vi "Runtime Test.vi"() -> ()   [LabVIEW 2014, in "DAQmx Watchdog tests.lvlib"]
uses:
  DAQmx Watchdog tests.lvlib
  module/execution/DAQmx Watchdog runtime.lvclass
  <vilib>/NI/Tag Bus/dictionary/data dictionary.lvclass/data dictionary.ctl
  <vilib>/NI/Tag Bus/dictionary/lookup polymorphs/locate Boolean.vi
  <vilib>/NI/Tag Bus/table/data polymorphs/read one/read Boolean.vi
  <vilib>/NI/Tag Bus/table/data polymorphs/write one/write Boolean.vi
  <vilib>/NI/Tag Bus/dictionary/search/find data index.vi
  <vilib>/NI/Tag Bus/dictionary/search/search string list.vi
  <vilib>/NI/Tag Bus/dictionary/tag not found.vi
  module/configuration/DAQmx Watchdog configuration.lvclass
  <vilib>/NI/Tag Bus/dictionary/data dictionary.lvclass
  <vilib>/NI/Tag Bus/table/data table.lvlib
panel:
  out "Expired?":bool
  out "input lookup error":errorcluster
  out "input error":errorcluster
  out "process result lookup error":errorcluster
  out "final error":errorcluster
  out "output error":errorcluster
  out "process error":errorcluster
  out "output lookup error":errorcluster
  out "process parameter  lookup error":errorcluster
  out "correct execution settings":bool
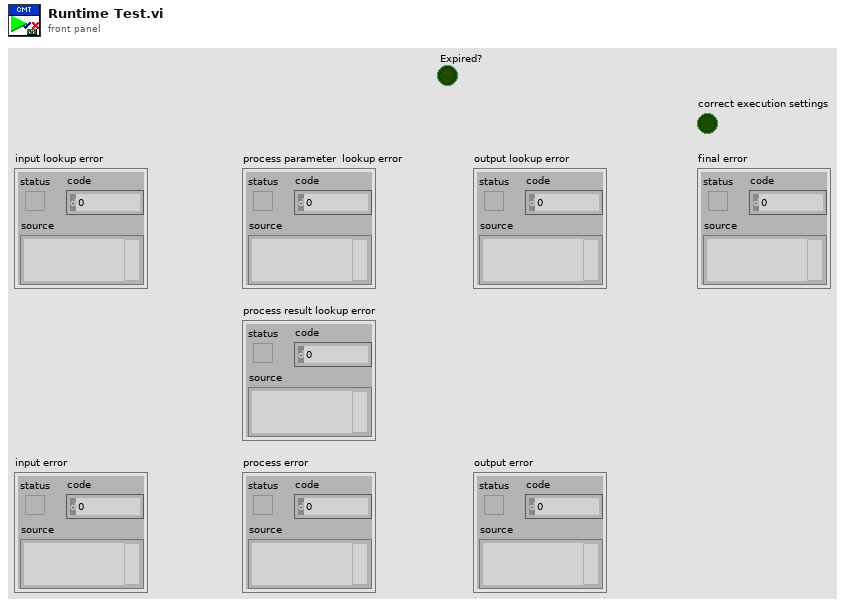
[diagram p1: front panel]
types:
  T1 = typedef "TBM channel.lvclass/data tables.ctl" = cluster{"input data":T2, "processing parameter":T2, "processing result":T2, "output data":T2}
  T2 = typedef "tag bus.lvlib/dictionary table pair.ctl" = cluster{"data dictionary":refnum<class "data dictionary.lvclass">, "data table":T3}
  T3 = typedef "tag bus.lvlib/data table.lvlib/data table.ctl" = cluster{"Double":dbl[], "Single":sgl[], "I64":i64[], "I32":i32[], "I16":i16[], "I8":i8[], "U64":u64[], "U32":u32[], "U16":u16[], "U8":u8[], "Boolean":bool[], "String":string[], "Array of Double":cluster{"DBL Array":dbl[]}[], "Array of Single":cluster{"SGL Array":sgl[]}[], "Array of I64":cluster{"I64 Array":i64[]}[], "Array of I32":cluster{"I32 Array":i32[]}[], "Array of I16":cluster{"I16 Array":i16[]}[], "Array of I8":cluster{"I8 Array":i8[]}[], "Array of U64":cluster{"U64 Array":u64[]}[], "Array of U32":cluster{"U32 Array":u32[]}[], "Array of U16":cluster{"U16 Array":u16[]}[], "Array of U8":cluster{"U8 Array":u8[]}[], "Array of Boolean":cluster{"Boolean Array":bool[]}[], "Array of String":cluster{"String Array":string[]}[]}
  T4 = typedef "TBM module execution interface.lvclass/execution settings.ctl" = cluster{"reads inputs":bool, "processes data":bool, "writes outputs":bool}
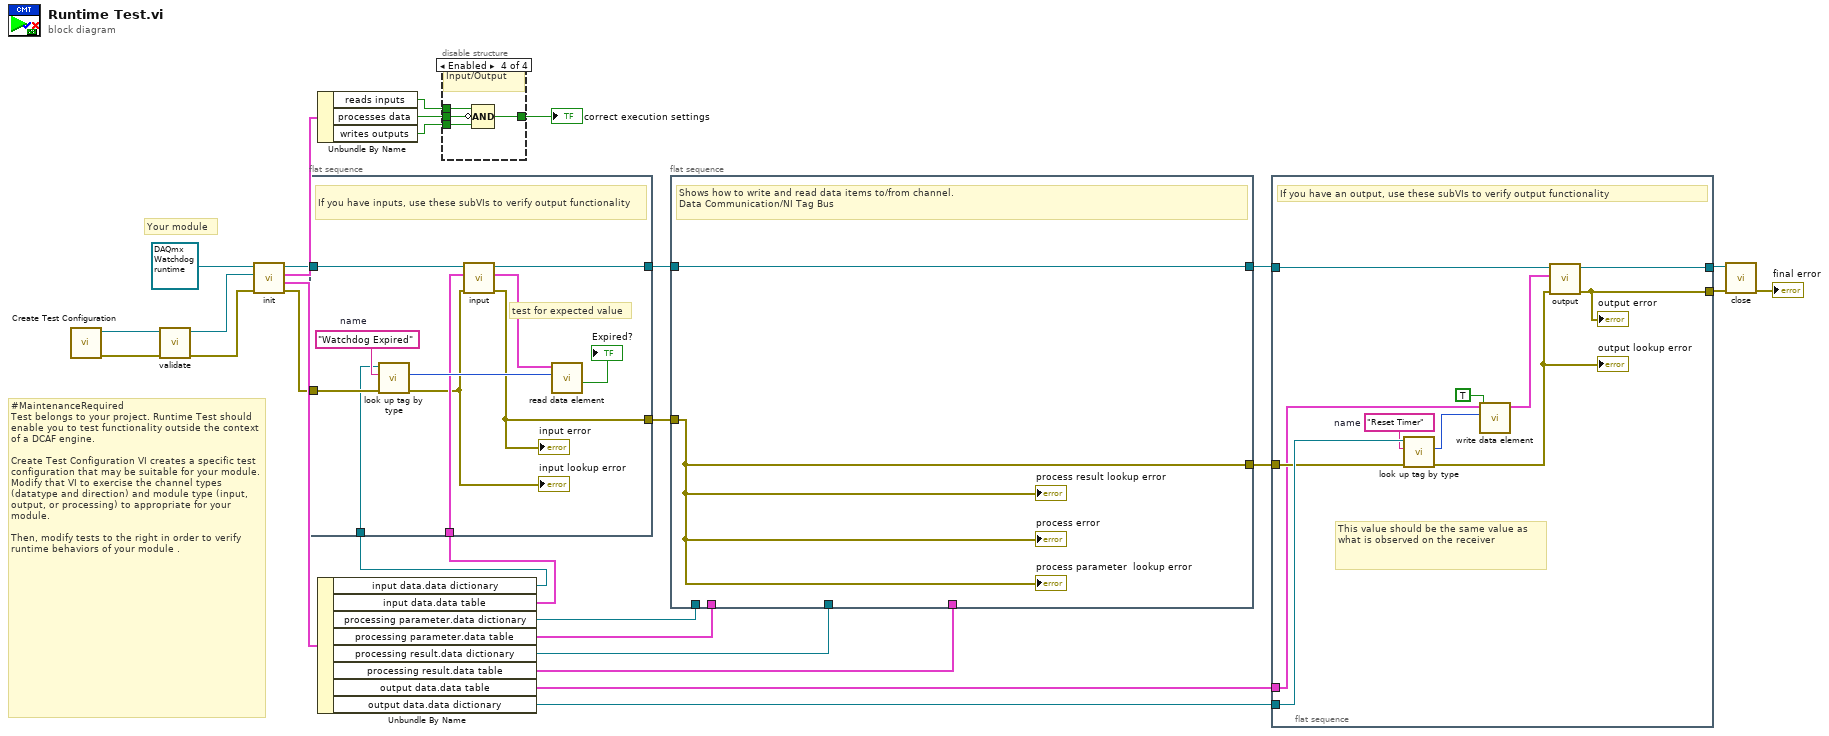
[diagram p0: block diagram]
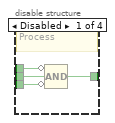
[diagram p2: hidden frame]
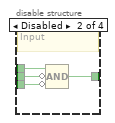
[diagram p3: hidden frame]
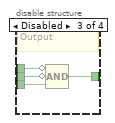
[diagram p4: hidden frame]
diagram:
  # "Your module"
  # "#MaintenanceRequired\nTest belongs to your project. Runtime Test should enable you to test functionality outside the context of a DCAF engine. \n\nCreate Test Configuration VI creates a specific test configuration that may be suitable for your module. Modify that VI to exercise the channel types (datatype and direction) and module type (input, output, or processing) to appropriate for your module. \n\nThen, modify tests to the right in order to verify runtime behaviors of your module ."
  n1 = call "Create Test Configuration.vi"() -> ("error out"=w9:errorcluster, "Module"=w11:refnum<class "DAQmx Watchdog configuration.lvclass">)  [unwired: 6 in, 4 out]
  n2 = call-dynamic "validate.vi"("error in"=w9, "fixed channel configuration in"=w11) -> ("error out"=w27:errorcluster, "fixed channel configuration out"=w28:refnum<class "DAQmx Watchdog configuration.lvclass">)  [unwired: 8 in]
  n3 = call-dynamic "init.vi"("error in"=w27, "TBM module configuration in"=w28, "fixed channel runtime in"=refnum<class "DAQmx Watchdog runtime.lvclass"> refnum ("user module")) -> ("error out"=w8:errorcluster, "data allocations"=w22:T1, "execution settings"=w26:T4, "fixed channel runtime out"=w6:refnum<class "DAQmx Watchdog runtime.lvclass">)  [unwired: 5 in]
  n4 = flat-sequence {
    tunnel: w8 -> [w36]
    tunnel: [w31] -> w7
    tunnel: w6 -> [w39]
    tunnel: [w38] -> w5
    tunnel: w4 -> [w35]
    tunnel: w1 -> [w32]
    frame #0 {
      w37 = "Watchdog Expired"  # name
      # "test for expected value"
      # "If you have inputs, use these subVIs to verify output functionality"
      n5 = call-poly <vilib>:"look up tag by type.vi"("error in"=w36, "name"=w37, "data dictionary in"=w35) -> ("error out"=w30:errorcluster, "index"=w33:i32)  [unwired: 6 in, 1 out]
      "input lookup error" <- w30
      n6 = call-dynamic "input.vi"("error in"=w30, "input allocation"=w32, "DAQmx Watchdog runtime in"=w39) -> ("error out"=w31:errorcluster, "input data"=w34:T3, "DAQmx Watchdog runtime out"=w38:refnum<class "DAQmx Watchdog runtime.lvclass">)  [unwired: 6 in]
      "input error" <- w31
      n7 = call-poly <vilib>:"read data element.vi"("index"=w33, "data table in"=w34) -> ("value"=→"Expired?":bool)  [unwired: 8 in, 1 out]
    }
  }
  n8 = Unbundle By Name(w26) -> ("reads inputs"=w24:bool, "processes data"=w12:bool, "writes outputs"=w25:bool)
  n9 = Unbundle By Name(w22) -> ("input data.data dictionary"=w4:refnum<class "data dictionary.lvclass">, "input data.data table"=w1:T3, "processing parameter.data dictionary"=w21:refnum<class "data dictionary.lvclass">, "processing parameter.data table"=w20:T3, "processing result.data dictionary"=w3:refnum<class "data dictionary.lvclass">, "processing result.data table"=w2:T3, "output data.data table"=w13:T3, "output data.data dictionary"=w19:refnum<class "data dictionary.lvclass">)
  n10 = disable-structure shown="Enabled" {
    disable-tunnel: w25 -> [w43 w47 w51 w55]
    disable-tunnel: w24 -> [w42 w46 w50 w54]
    disable-tunnel: [w41 w45 w49 w53] -> w23
    disable-tunnel: w12 -> [w40 w44 w48 w52]
    frame Disabled {
      # "Process"
      n11 = Compound Arithmetic op=AND(invert w42, w40, invert w43) -> (w41:bool)
    }
    frame Disabled {
      # "Input"
      n12 = Compound Arithmetic op=AND(w46, invert w44, invert w47) -> (w45:bool)
    }
    frame Disabled {
      # "Output"
      n13 = Compound Arithmetic op=AND(invert w50, invert w48, w51) -> (w49:bool)
    }
    frame Enabled {
      # "Input/Output"
      n14 = Compound Arithmetic op=AND(w54, invert w52, w55) -> (w53:bool)
    }
  }
  "correct execution settings" <- w23
  n15 = flat-sequence {
    tunnel: w21 -> [_]
    tunnel: w7 -> [w56]
    tunnel: w20 -> [_]
    tunnel: [w57] -> w15
    tunnel: [w56] -> w14
    tunnel: w5 -> [w57]
    tunnel: w3 -> [_]
    tunnel: w2 -> [_]
    frame #0 {
      # "Shows how to write and read data items to/from channel.\nData Communication/NI Tag Bus"
      "process parameter  lookup error" <- w56
      "process error" <- w56
      "process result lookup error" <- w56
    }
  }
  n16 = flat-sequence {
    tunnel: w19 -> [w68]
    tunnel: [w65] -> w18
    tunnel: [w64] -> w17
    tunnel: w15 -> [w63]
    tunnel: w14 -> [w62]
    tunnel: w13 -> [w61]
    frame #0 {
      w59 = "Reset Timer"  # name
      # "This value should be the same value as what is observed on the receiver"
      # "If you have an output, use these subVIs to verify output functionality"
      n17 = call-poly <vilib>:"look up tag by type.vi"("error in"=w62, "name"=w59, "data dictionary in"=w68) -> ("error out"=w60:errorcluster, "index"=w67:i32)  [unwired: 6 in, 1 out]
      "output lookup error" <- w60
      n18 = call-poly <vilib>:"write data element.vi"("value"=TRUE, "index"=w67, "data table in"=w61) -> ("data table out"=w66:T3)  [unwired: 8 in]
      n19 = call-dynamic "output.vi"("error in"=w60, "output data"=w66, "DAQmx Watchdog runtime in"=w63) -> ("error out"=w64:errorcluster, "DAQmx Watchdog runtime out"=w65:refnum<class "DAQmx Watchdog runtime.lvclass">)  [unwired: 6 in, 1 out]
      "output error" <- w64
    }
  }
  n20 = call-dynamic "close.vi"("error in"=w17, "module in"=w18) -> ("error out"=→"final error":errorcluster)  [unwired: 9 in]
